vi "randn_approximation.vi"(1 "normalize to +/-1 (True)":bool=TRUE, 2 "N":i32) -> (0 "randn() vector":dbl[](array[numeric]))   [LabVIEW 2020]
doc: "Normal distribution random number generator (aproximation)."
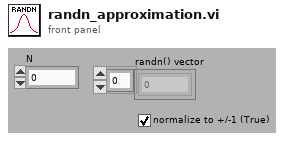
[diagram p1: front panel]
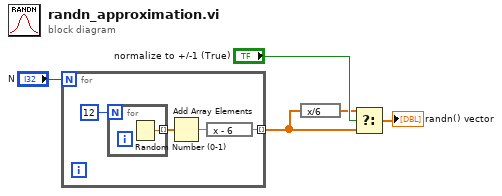
[diagram p0: block diagram]
diagram:
  n1 = for {
    N: "N" -> [_]
    tunnel: [w6] -> w2 mode=indexing
    n2 = for {
      N: 12 -> [_]
      tunnel: [w10] -> w8 mode=indexing
      n3 = Random Number (0-1)() -> (number: 0 to 1=w10:dbl)
    }
    n4 = Add Array Elements(numeric array=w8) -> (sum=w7:dbl)
    n5 = expression code="x - 6"(w7) -> (w6:dbl)
  }
  n6 = expression code="x/6"(w2) -> (w3:dbl[])
  n7 = Select(t=w3, s="normalize to +/-1 (True)", f=w2) -> (s? t:f=→"randn() vector":dbl[])
